vi "Get S-Param Mag.vi"(4 "error in":errorcluster, 6 "Trace Name":T2, 7 "Data in":T1 {"LogStartTime" format="%<%x %.3X>T"}) -> (0 "error out":errorcluster, 1 "Graph":cluster{"Array":dbl[], "Array":dbl[]}, 2 "size(s)":i32[](array[numeric]), 3 "Data Out":T1 {"LogStartTime" format="%<%x %.3X>T"})   [LabVIEW 2023]
uses:
  controls/UI Data.ctl
  <vilib>/NI/Modbus Library/API/Master/Modbus Master.lvclass
  LibreVNA/LibreVNA.lvclass
  LibreVNA/Types/Trace Enum.ctl
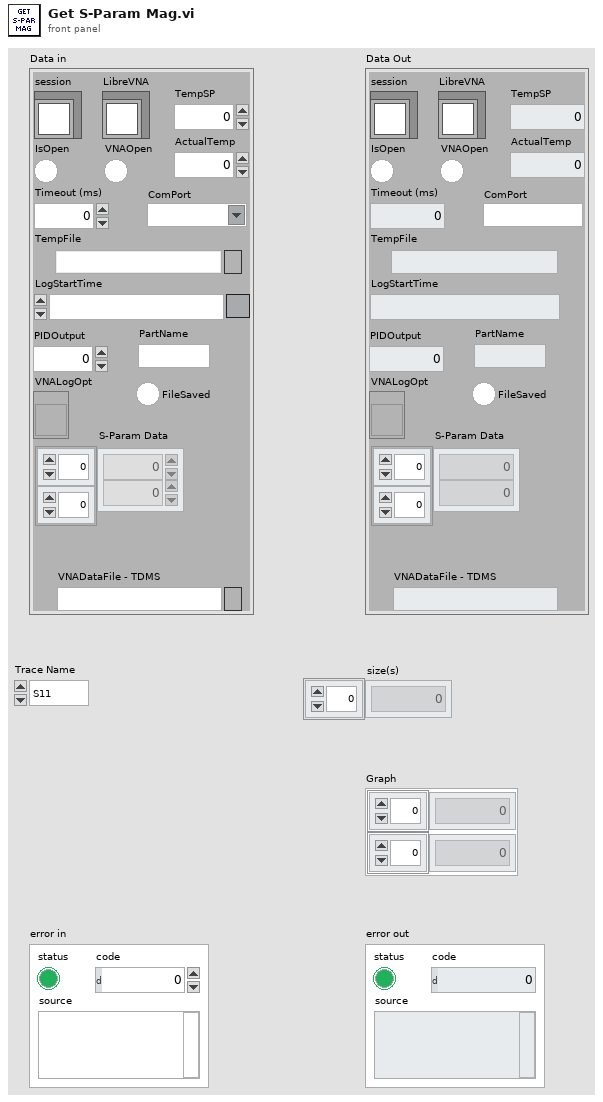
[diagram p1: front panel]
types:
  T1 = typedef "UI Data.ctl" = cluster{"session":refnum<class "Modbus Master.lvclass">, "IsOpen":bool, "Timeout (ms)":i32, "TempFile":path, "LogStartTime":timestamp, "LibreVNA":refnum<class "LibreVNA.lvclass">, "VNAOpen":bool, "TempSP":dbl, "ActualTemp":dbl, "FileSaved":bool, "PIDOutput":dbl, "VNALogOpt":refnum<vi>, "PartName":string, "ComPort":refnum<visa-resource-name>, "S-Param Data":dbl[][], "VNADataFile - TDMS":path}
  T2 = typedef "LibreVNA.lvclass/Trace Enum.ctl" = enum16{"S11", "S12", "S21", "S22"}
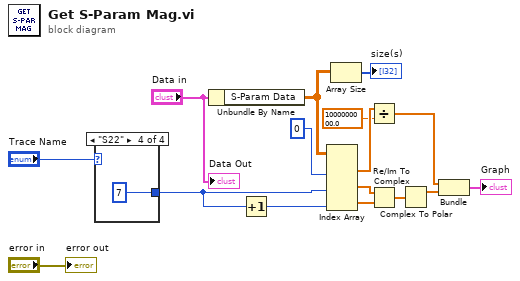
[diagram p0: block diagram]
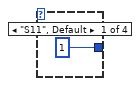
[diagram p2: hidden frame]
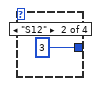
[diagram p3: hidden frame]
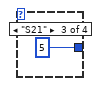
[diagram p4: hidden frame]
diagram:
  n1 = case shown="\"S22\"" "Trace Name" {
    tunnel: [1 ("disabled index (col)") 3 ("disabled index (col)") 5 ("disabled index (col)") 7 ("disabled index (col)")] -> w13
    frame "S11", Default {
    }
    frame "S12" {
    }
    frame "S21" {
    }
    frame "S22" {
    }
  }
  n2 = Unbundle By Name("Data in") -> ("S-Param Data"=w2:dbl[][])
  n3 = Increment(x=w13) -> (x+1=w12:i32)
  n4 = Index Array(array=w2, index (col) #1=0 ("disabled index (col)"), index (col) #2=w13, index (col) #3=w12) -> (element #1=w8:dbl[], element #2=w6:dbl[], element #3=w5:dbl[])  [unwired: 3 in]
  n5 = Array Size(array=w2) -> (size(s)=→"size(s)":i32[])
  n6 = Divide(x=w8, y=1000000000.0) -> (x/y=w9:dbl[])
  n7 = Re/Im To Complex(1:w5, 2:w6) -> (0:w11:cdb[])
  n8 = Complex To Polar(r * e^(i*theta)=w11) -> (r=w10:dbl[])  [unwired: 1 out]
  n9 = Bundle(w9, w10) -> (→"Graph":cluster{dbl[], dbl[]})  [unwired: 1 in]
  "Data Out" <- "Data in"
  "error out" <- "error in"
